vi "Retry Call Measure.vi"(8 "error in (no error)":errorcluster, 10 "Data In":T1, 11 "Message Queue":refnum<queue>) -> (0 "error out":errorcluster, 2 "data out":T1, 3 "dup Message Queue":refnum<queue>)   [LabVIEW 2020, in "InstrumentStudioPlugin.lvlib"]
uses:
  InstrumentStudioPlugin.lvlib
  Message Queue/Message Cluster.ctl
  Measurement Client Wrapper/Measurement Client Wrapper.lvclass
  controls/Data.ctl
  Message Queue/Enqueue Message (Single).vi
  Message Queue/Message Queue.lvlib
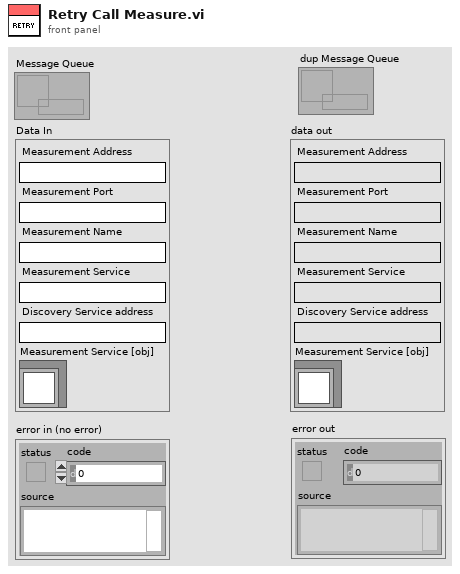
[diagram p1: front panel]
types:
  T1 = typedef "InstrumentStudioPlugin.lvlib/Data.ctl" = cluster{"Measurement Address":string, "Measurement Port":string, "Measurement Name":string, "Measurement Service":string, "Discovery Service address":string, "Measurement Service [obj]":refnum<class "Measurement Client Wrapper.lvclass">}
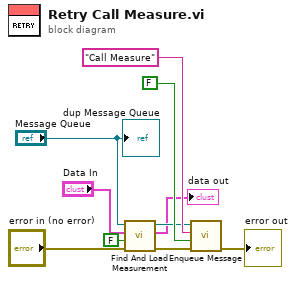
[diagram p0: block diagram]
diagram:
  n1 = call "Find And Load Measurement.vi"("error in (no error)"="error in (no error)", "Reset Defaults"=FALSE, "data in"="Data In", "Queue in"="Message Queue") -> ("error out"=w4:errorcluster, "data out"=→"data out":T1, "dup Queue in"=w7:refnum<queue>)  [unwired: 5 in]
  n2 = call-poly "Enqueue Message.vi"("error in (no error)"=w4, "Message Data"=FALSE, "Message"="Call Measure", "Message Queue"=w7) -> ("error out"=→"error out":errorcluster)  [unwired: 6 in, 1 out]
  "dup Message Queue" <- "Message Queue"
